vi "Actor Core.vi"(8 "error in":errorcluster, 11 "Signal Acquisition in":refnum<class "Signal Acquisition.lvclass">) -> (0 "error out":errorcluster, 3 "Actor out":refnum<class "Actor.lvclass">)   [LabVIEW 2022 SP3, in "Signal Acquisition.lvlib" / "Signal Acquisition.lvclass"]
doc: "(<B>Filename</B>: Actor Framework.lvlib:Actor.lvclass:Actor Core.vi)\n\nReceives messages to the actor, reacts to them, and initiates any error handling that may shut the actor down.\n\nDescendant classes may override this VI to append parallel tasks for the actor to complete while it handles messages. Overrides use the Call Parent Class Method node."
uses:
  Signal Acquisition.lvclass
  C:/Program Files/National Instruments/LabVIEW 2022/vi.lib/ActorFramework/Actor/Actor.lvclass
  <vilib>/ActorFramework/Actor/Actor.lvclass
  <vilib>/NI/Modbus Library/API/Master/Modbus Master.lvclass
  Controls/States.ctl
  Signal Acquisition.lvclass/Signal Acquisition.ctl
  <vilib>/ActorFramework/Actor/Actor.lvclass/Actor.ctl
  <vilib>/ActorFramework/Message Enqueuer/Message Enqueuer.lvclass/Message Enqueuer.ctl
  Controller -- Sig Acq Interface Messages/Incoming Bit Msg/Incoming Bit Msg.lvclass/Incoming Bit Msg.ctl
  <vilib>/ActorFramework/Message Enqueuer/Init from Existing Queue.vi
  <vilib>/ActorFramework/Message Enqueuer/Enqueue.vi
  Controller -- Sig Acq Interface Messages/Incoming Bit Msg/Incoming Bit Msg.lvclass
  C:/Program Files/National Instruments/LabVIEW 2022/vi.lib/ActorFramework/Message/Message.lvclass
  <vilib>/ActorFramework/Stop Msg/Stop Msg.lvclass
  <vilib>/ActorFramework/Message Priority Queue/Priority Enqueue.vi
  <vilib>/NI/Modbus Library/API/Wrapper/Create Serial Master.vi
  <vilib>/ActorFramework/Message Enqueuer/Message Enqueuer.lvclass
  Signal Acquisition.lvlib
  <vilib>/NI/Modbus Library/API/Wrapper/API Main.lvlib
  Controller/Controller Messages/Incoming Bit Msg/Incoming Bit Msg.lvclass
panel:
  in  "Signal Parameters":T1
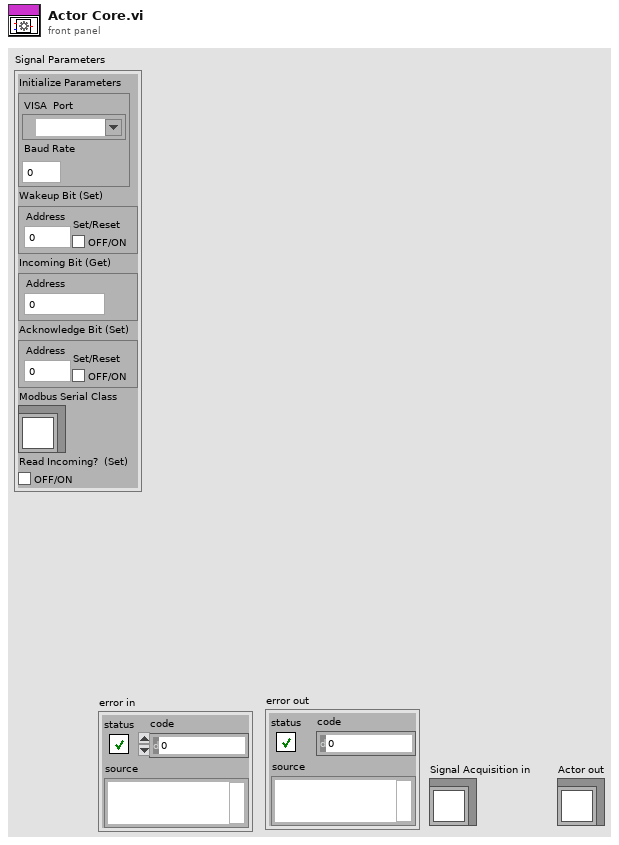
[diagram p1: front panel]
types:
  T1 = cluster{"Initialize Parameters":cluster{"VISA  Port":refnum<visa-resource-name>, "Baud Rate":u32}, "Wakeup Bit (Set)":cluster{"Address":u16, "Set/Reset":bool}, "Incoming Bit (Get)":cluster{"Address":u16}, "Acknowledge Bit (Set)":cluster{"Address":u16, "Set/Reset":bool}, "Modbus Serial Class":refnum<class "Modbus Master.lvclass">, "Read Incoming?  (Set)":bool}
  T2 = typedef "Signal Acquisition.lvlib/States.ctl" = enum16{"Poll", "Initialize", "Read Start bit", "Read End bit", "Send Start", "Send Ack", "Error", "Exit"}
  T3 = cluster{"Stop Actor":refnum<user-event>, "Wakeup Bit Event":refnum<user-event>, "Acknowledge Bit Event":refnum<user-event>, "Incoming Bit event":refnum<user-event>}
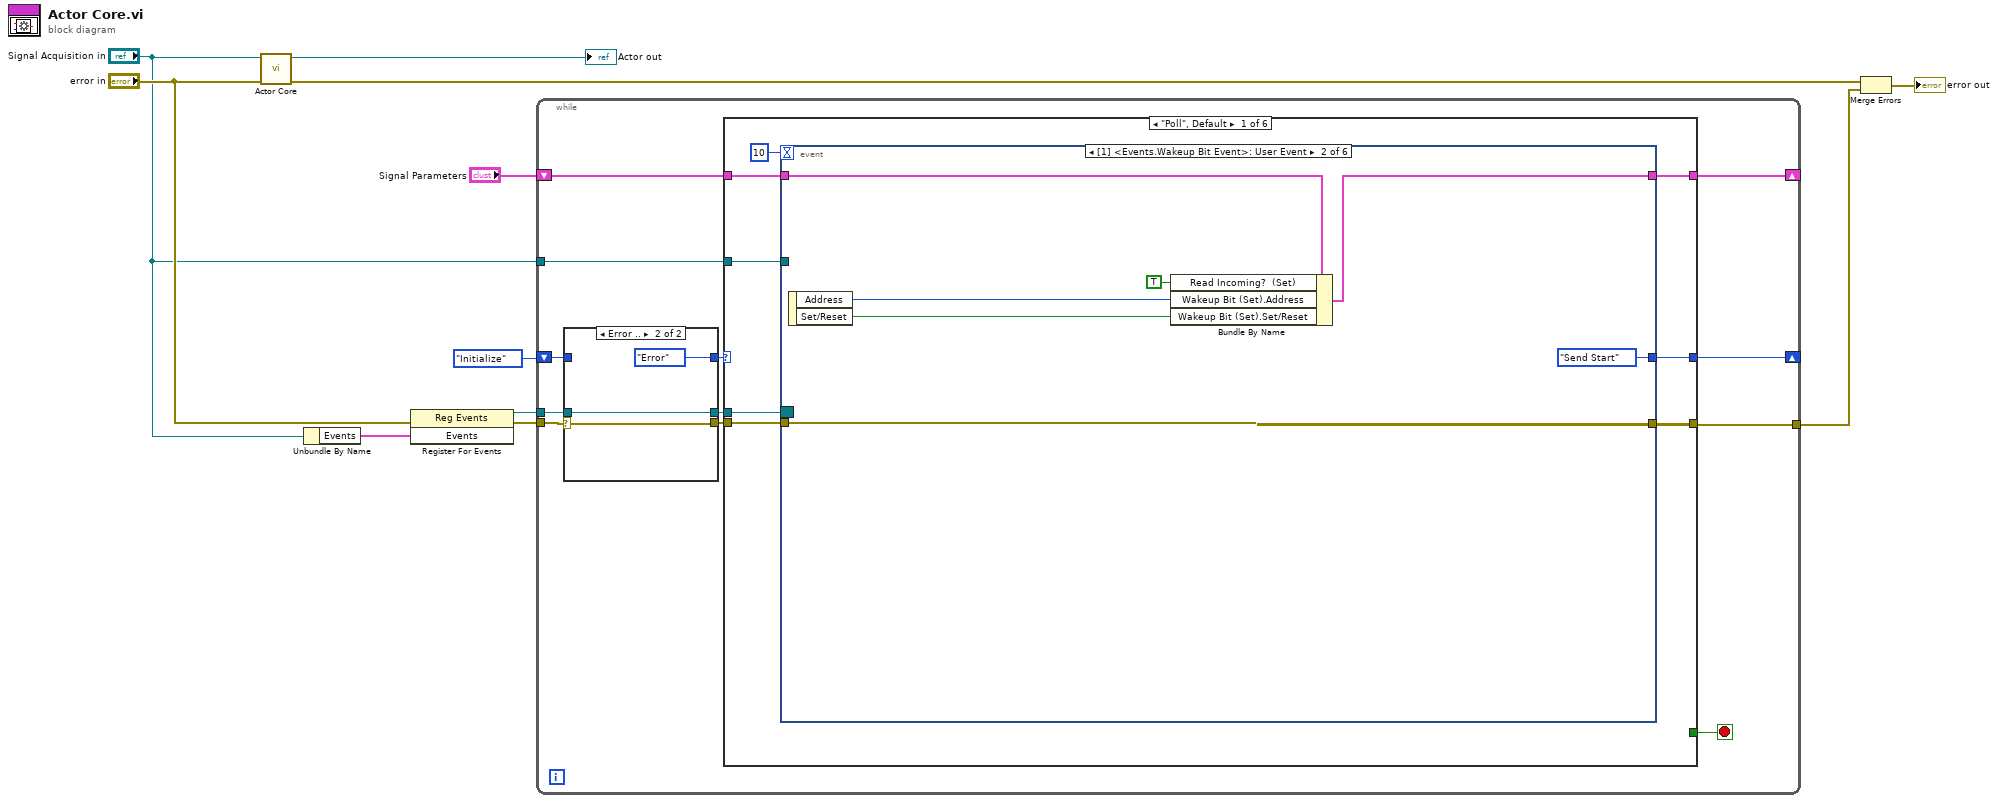
[diagram p0: block diagram]
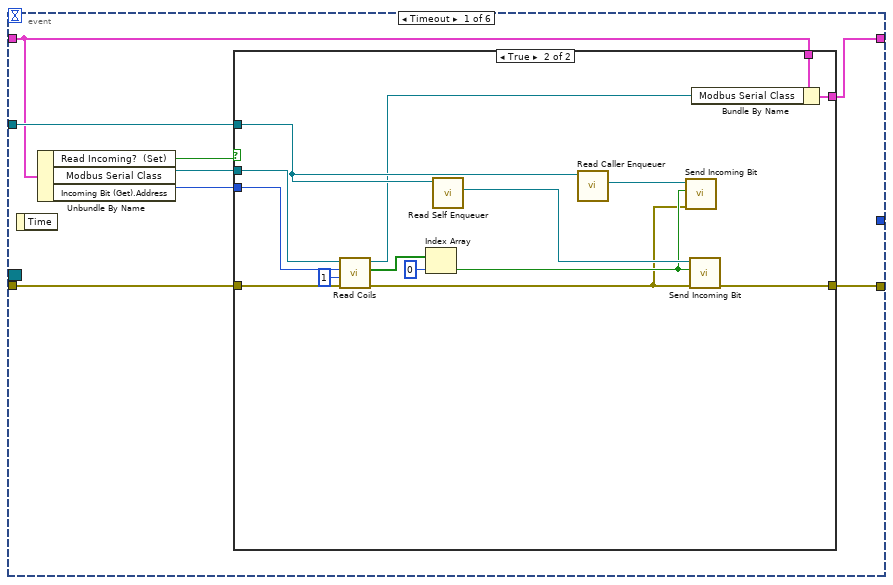
[diagram p3: hidden frame]
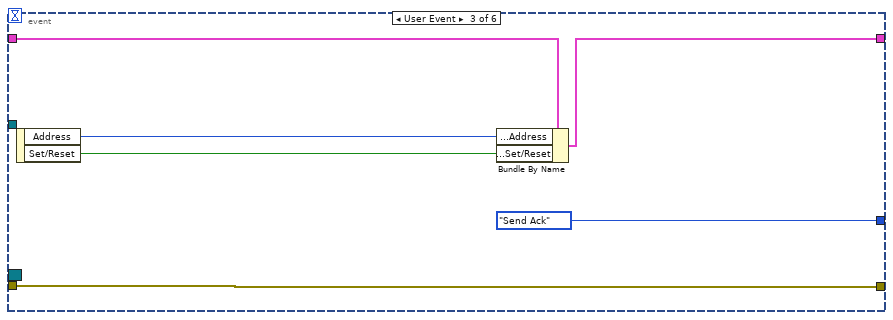
[diagram p5: hidden frame]
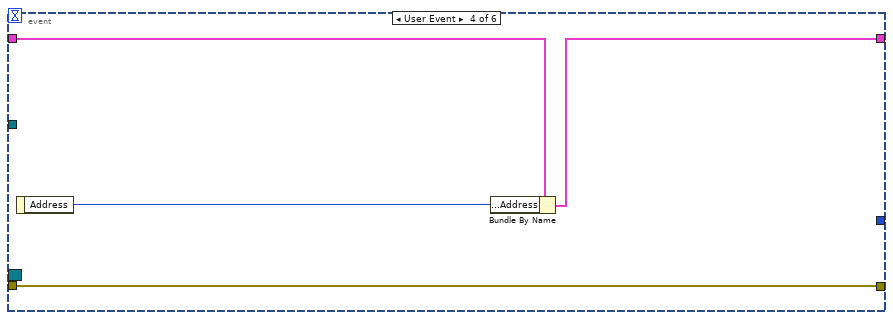
[diagram p6: hidden frame]
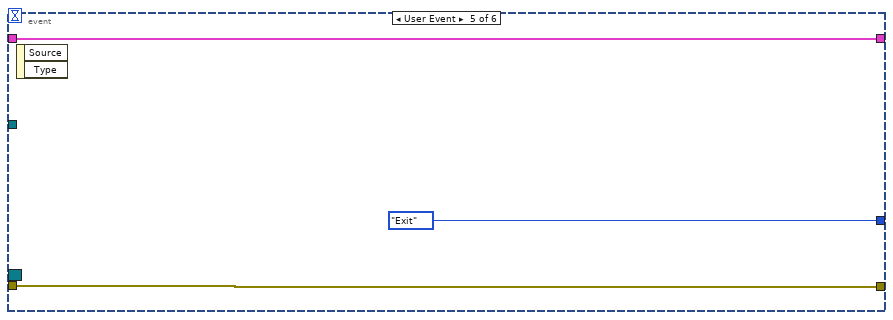
[diagram p7: hidden frame]
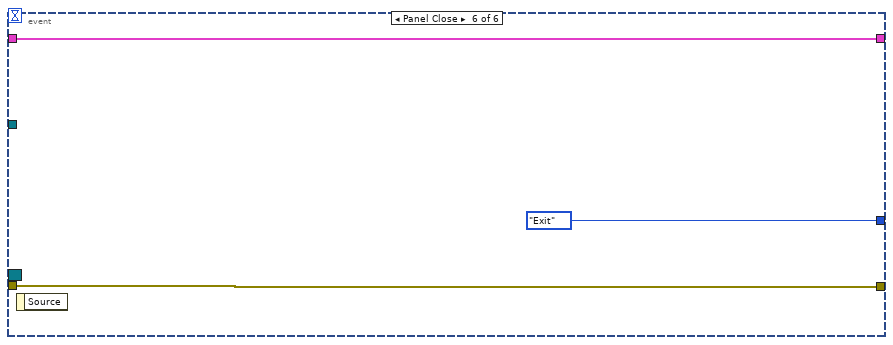
[diagram p8: hidden frame]
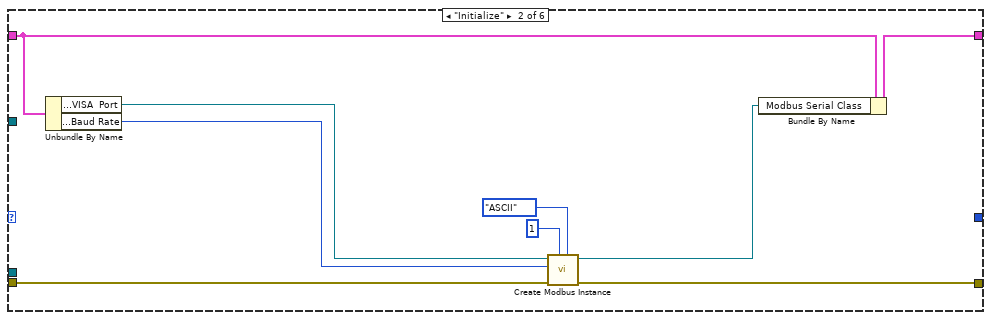
[diagram p9: hidden frame]
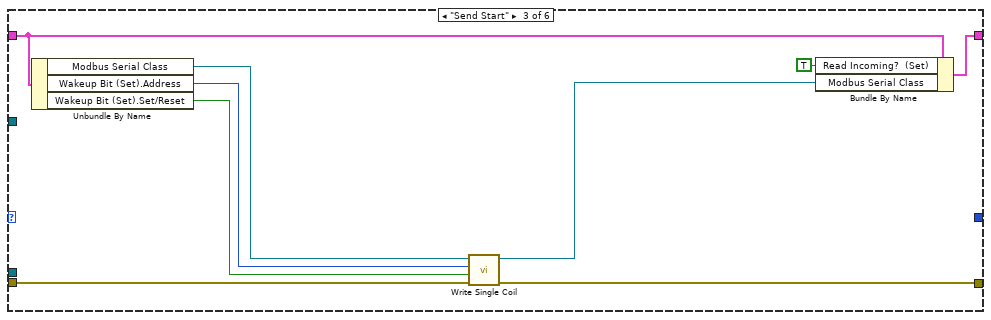
[diagram p10: hidden frame]
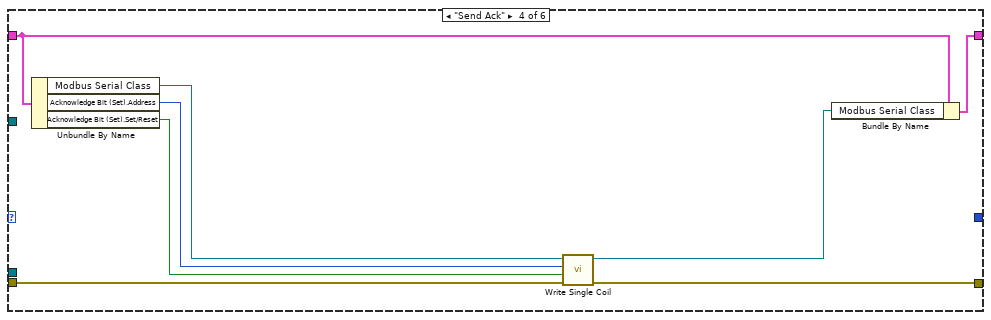
[diagram p11: hidden frame]
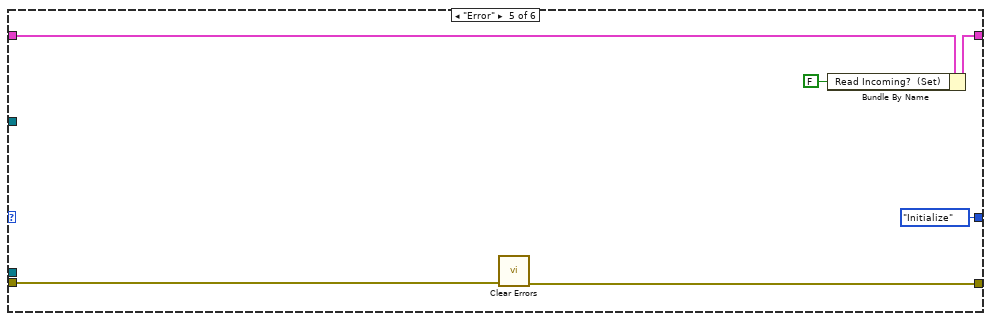
[diagram p12: hidden frame]
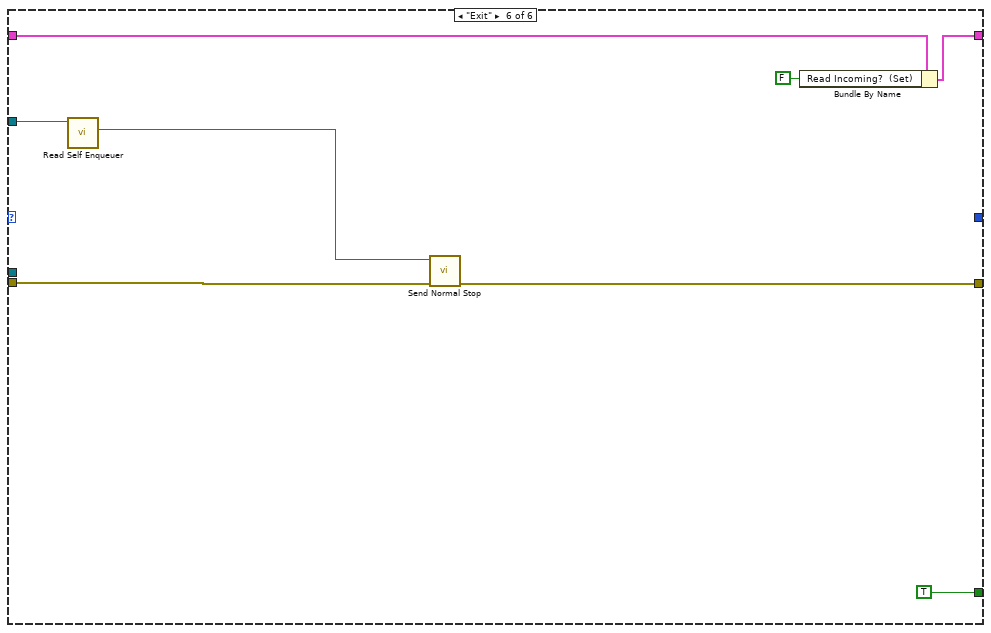
[diagram p13: hidden frame]
diagram:
  n1 = call-parent "Actor Core.vi"("error in"="error in", "Actor in"="Signal Acquisition in") -> ("error out"=w9:errorcluster, "Actor out"=→"Actor out":refnum<class "Actor.lvclass">)  [unwired: 8 in]
  n2 = Unbundle By Name("Signal Acquisition in") -> ("Events"=w3:T3)
  n3 = register-events(error in="error in", w3) -> (reference out=w5:refnum<event-registration>, error out=w6:errorcluster)  [unwired: 1 in]
  n4 = while {
    shift-right: [w22] -> _
    shift-left: States."Initialize" -> [w16]
    tunnel: w6 -> [w17]
    tunnel: [w23] -> w7
    tunnel: w5 -> [w19]
    shift-right: [w13] -> _
    shift-left: "Signal Parameters" -> [w14]
    tunnel: "Signal Acquisition in" -> [w12]
    stop <- w21 stop-if-true
    n5 = case shown="Error .." w17 {
      selector: w17 -> [w25 w27]
      tunnel: [w25 w27] -> w20
      tunnel: w19 -> [w26 w28]
      tunnel: [w26 w28] -> w18
      tunnel: w16 -> [w24 _]
      tunnel: [w24 States."Error"] -> w15
      frame No Error {
      }
      frame Error {
      }
    }
    n6 = case shown="\"Poll\", Default" w15 {
      tunnel: w20 -> [w36 w94 w103 w109 w117 w123]
      tunnel: [w35 w93 w102 w108 w116 w124] -> w23
      tunnel: [w34 _ _ _ States."Initialize" _] -> w22
      tunnel: [_ _ _ _ _ TRUE] -> w21
      tunnel: w18 -> [w33 _ _ _ _ _]
      tunnel: w14 -> [w32 w92 w98 w110 w115 w119]
      tunnel: [w31 w89 w97 w111 w114 w118] -> w13
      tunnel: w12 -> [w30 _ _ _ _ w122]
      frame "Poll", Default {
        n7 = event shown="[1] <Events.Wakeup Bit Event>: User Event" {
          selector: w33 -> [_ _ _ _ _ _]
          dyn-events: _ -> [_ _ _ _ _ _]
          timeout: 10 -> [_ _ _ _ _ _]
          tunnel: w36 -> [w45 w64 w75 w78 w81 w84]
          tunnel: [w44 w64 w75 w78 w81 w84] -> w35
          tunnel: [_ States."Send Start" States."Send Ack" _ States."Exit" States."Exit"] -> w34
          tunnel: w32 -> [w39 w69 w73 w79 w80 w83]
          tunnel: [w38 w67 w72 w77 w80 w83] -> w31
          tunnel: w30 -> [w40 _ _ _ _ _]
          event Timeout {
            n8 = event-data() -> ()  [unwired: 1 in, 1 out]
            n9 = Unbundle By Name(w39) -> ("Read Incoming?  (Set)"=w41:bool, "Modbus Serial Class"=w42:refnum<class "Modbus Master.lvclass">, "Incoming Bit (Get).Address"=w43:u16)
            n10 = case shown="True" w41 {
              tunnel: w45 -> [w47 w62]
              tunnel: [w47 w55] -> w44
              tunnel: w43 -> [_ w61]
              tunnel: w42 -> [_ w60]
              tunnel: w40 -> [_ w54]
              tunnel: w39 -> [w46 w50]
              tunnel: [w46 w49] -> w38
              frame False {
              }
              frame True {
                n11 = call-dynamic "Read Coils.vi"("error in"=w62, "number of inputs"=u16 1, "starting address"=w61, "Modbus master in"=w60) -> ("error out"=w51:errorcluster, "coils"=w58:bool[], "Modbus master out"=w48:refnum<class "Modbus Master.lvclass">)  [unwired: 5 in]
                n12 = Index Array(array=w58, index=0) -> (element=w53:bool)
                n13 = call <vilib>:"Read Self Enqueuer.vi"("Actor"=w54) -> ("Self Enqueuer"=w56:refnum<class "Message Enqueuer.lvclass">)  [unwired: 10 in]
                n14 = call <vilib>:"Read Caller Enqueuer.vi"("Actor"=w54) -> ("Caller Enqueuer"=w52:refnum<class "Message Enqueuer.lvclass">)  [unwired: 10 in]
                n15 = call "Send Incoming Bit.vi"("error in (no error)"=w51, "Set/Reset"=w53, "Message Enqueuer"=w52) -> ()  [unwired: 7 in, 2 out]
                n16 = call "Send Incoming Bit.vi"("error in (no error)"=w51, "Set/Reset"=w53, "Message Enqueuer"=w56) -> ("error out"=w55:errorcluster)  [unwired: 7 in, 1 out]
                n17 = Bundle By Name(cluster=w50, "Modbus Serial Class"=w48) -> (w49:T1)
              }
            }
          }
          event User Event {
            n18 = event-data() -> ("Address"=w66:u16, "Set/Reset"=w65:bool)  [unwired: 1 in]
            n19 = Bundle By Name(cluster=w69, "Read Incoming?  (Set)"=TRUE, "Wakeup Bit (Set).Address"=w66, "Wakeup Bit (Set).Set/Reset"=w65) -> (w67:T1)
          }
          event User Event {
            n20 = event-data() -> ("Address"=w70:u16, "Set/Reset"=w71:bool)  [unwired: 1 in]
            n21 = Bundle By Name(cluster=w73, "Acknowledge Bit (Set).Address"=w70, "Acknowledge Bit (Set).Set/Reset"=w71) -> (w72:T1)
          }
          event User Event {
            n22 = event-data() -> ("Address"=w76:u16)  [unwired: 1 in]
            n23 = Bundle By Name(cluster=w79, "Incoming Bit (Get).Address"=w76) -> (w77:T1)
          }
          event User Event {
            n24 = event-data() -> ()  [unwired: 1 in, 2 out]
          }
          event Panel Close {
            n25 = event-data() -> ()  [unwired: 1 in, 1 out]
          }
        }
      }
      frame "Initialize" {
        n26 = Unbundle By Name(w92) -> ("Initialize Parameters.VISA  Port"=w90:refnum<visa-resource-name>, "Initialize Parameters.Baud Rate"=w91:u32)
        n27 = call-poly <vilib>:"Create Modbus Instance.vi"("serial type"=enum16{"RTU", "ASCII"}."ASCII", "unit ID"=u8 1, "error in"=w94, "baud rate"=w91, "VISA resource name"=w90) -> ("error out"=w93:errorcluster, "serial master instance"=w88:refnum<class "Modbus Master.lvclass">)  [unwired: 5 in]
        n28 = Bundle By Name(cluster=w92, "Modbus Serial Class"=w88) -> (w89:T1)
      }
      frame "Send Start" {
        n29 = Unbundle By Name(w98) -> ("Modbus Serial Class"=w100:refnum<class "Modbus Master.lvclass">, "Wakeup Bit (Set).Address"=w101:u16, "Wakeup Bit (Set).Set/Reset"=w99:bool)
        n30 = call-dynamic "Write Single Coil.vi"("error in"=w103, "coil to write"=w99, "address"=w101, "Modbus master in"=w100) -> ("error out"=w102:errorcluster, "Modbus master out"=w96:refnum<class "Modbus Master.lvclass">)  [unwired: 6 in]
        n31 = Bundle By Name(cluster=w98, "Read Incoming?  (Set)"=TRUE ("Read Ack?  (Set)"), "Modbus Serial Class"=w96) -> (w97:T1)
      }
      frame "Send Ack" {
        n32 = Unbundle By Name(w110) -> ("Modbus Serial Class"=w107:refnum<class "Modbus Master.lvclass">, "Acknowledge Bit (Set).Address"=w104:u16, "Acknowledge Bit (Set).Set/Reset"=w105:bool)
        n33 = call-dynamic "Write Single Coil.vi"("error in"=w109, "coil to write"=w105, "address"=w104, "Modbus master in"=w107) -> ("error out"=w108:errorcluster, "Modbus master out"=w106:refnum<class "Modbus Master.lvclass">)  [unwired: 6 in]
        n34 = Bundle By Name(cluster=w110, "Modbus Serial Class"=w106) -> (w111:T1)
      }
      frame "Error" {
        n35 = call <vilib>:"Clear Errors.vi"("error in (no error)"=w117) -> ("error out"=w116:errorcluster)  [unwired: 5 in, 1 out]
        n36 = Bundle By Name(cluster=w115, "Read Incoming?  (Set)"=FALSE) -> (w114:T1)
      }
      frame "Exit" {
        n37 = call <vilib>:"Read Self Enqueuer.vi"("Actor"=w122) -> ("Self Enqueuer"=w121:refnum<class "Message Enqueuer.lvclass">)  [unwired: 10 in]
        n38 = call <vilib>:"Send Normal Stop.vi"("error in (no error)"=w123, "Message Enqueuer"=w121) -> ("error out"=w124:errorcluster)  [unwired: 9 in]
        n39 = Bundle By Name(cluster=w119, "Read Incoming?  (Set)"=FALSE) -> (w118:T1)
      }
    }
  }
  n40 = Merge Errors(w9, w7) -> (→"error out":errorcluster)
